vi "Sequence.Status.Replace.vi"(0 "old status":T1, 1 "new status (Done)":T1=enum."Done") -> (2 "status out":T1)   [LabVIEW 2016]
uses:
  Sequence.Step.Status.ctl
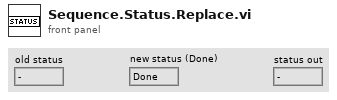
[diagram p1: front panel]
types:
  T1 = typedef "Sequence.Step.Status.ctl" = enum16{"-", "Pending", "Running", "Skipped", "Passed", "Failed", "Done", "Error", "Aborted", "Stopped"}
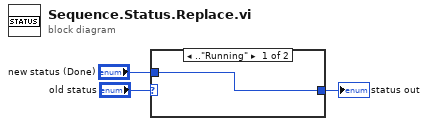
[diagram p0: block diagram]
diagram:
  n1 = case shown="..\"Running\"" "old status" {
    selector: "old status" -> [_ w5]
    tunnel: [w4 w5] -> w3
    tunnel: "new status (Done)" -> [w4 _]
    frame .."Running" {
    }
    frame Default {
    }
  }
  "status out" <- w3
